vi "APU + 4 Digital Patterns.vi"() -> ()   [LabVIEW 2013]
uses:
  IP Source/Digital Pattern Generation/Load Input.ctl
  IP Source/Digital Pattern Generation/Input.ctl
  IP Source/Digital Pattern Generation/Settings.ctl
  IP Source/APU/Settings.ctl
  IP Source/APU/Input.ctl
  IP Source/APU/Output.ctl
  IP Source/Version Token.ctl
  IP Source/APU/Shared Settings.ctl
  <vilib>/Platform/TimedLoop/XDataNode/timing_clust.ctl
  <vilib>/Platform/TimedLoop/XDataNode/nitl_modes.ctl
  <vilib>/Platform/TimedLoop/XDataNode/wakeup.ctl
  <vilib>/rvi/DataTransferAndStorage/Container/Common/niFpgaContainerGetUniqueNameForEmu.vi
  <vilib>/rvi/DataTransferAndStorage/Container/Common/niFpgaContainerSetEmuInfo.vi
  <vilib>/rvi/eio/common/nirviEmuReportErrorAndStop.vi
  <vilib>/rvi/Emulation/niFpgaSctlEmulationGetInTimedLoop.vi
  <vilib>/rvi/Emulation/niFpgaEmulationReportErrorSimple.vi
  <vilib>/rvi/Emulation/niFpgaGetClockAttributes.vi
  <vilib>/rvi/Emulation/niFpgaCriticalErrorInLSC.vi
  <vilib>/rvi/eio/common/nirviEmuTemplateMethod_errors.vi
  <vilib>/Platform/TimedLoop/XDataNode/XDataNode.xnode
  <vilib>/rvi/LocalResourceManager/LocalResourceManager.xnode
  <vilib>/eio/EIONode/EIONode.xnode
  <vilib>/Platform/TimedLoop/XDataNode/XDNodeRunTimeDep.lvlib
  IP Source/Digital Pattern Generation/Digital Pattern Generation.lvlib
  IP Source/APU/APU.lvlib
  IP Source/Engine Simulation Toolkit.lvlib
panel:
  in  "shared settings.my apu":T1 {"start" format="%#.15g"}
  in  "go.my apu":bool
  in  "est.version":T2
  out "output.my apu":T3 caption="output"
  in  "input.my apu":T4={"desired speed"=0.0, "reset"=TRUE} caption="input"
  in  "settings.my apu":T5 caption="settings"
  in  "input.Pattern 3":T6
  in  "settings.Pattern 3":T7
  in  "input.Pattern 4":T6
  in  "settings.Pattern 4":T7
  in  "input.Pattern 2":T6
  in  "settings.Pattern 2":T7
  in  "settings.Pattern 1":T7
  in  "input.Pattern 1":T6
  in  "load input.Pattern 4":T8
  in  "load input.Pattern 3":T8
  in  "load input.Pattern 2":T8
  in  "load input.Pattern 1":T8
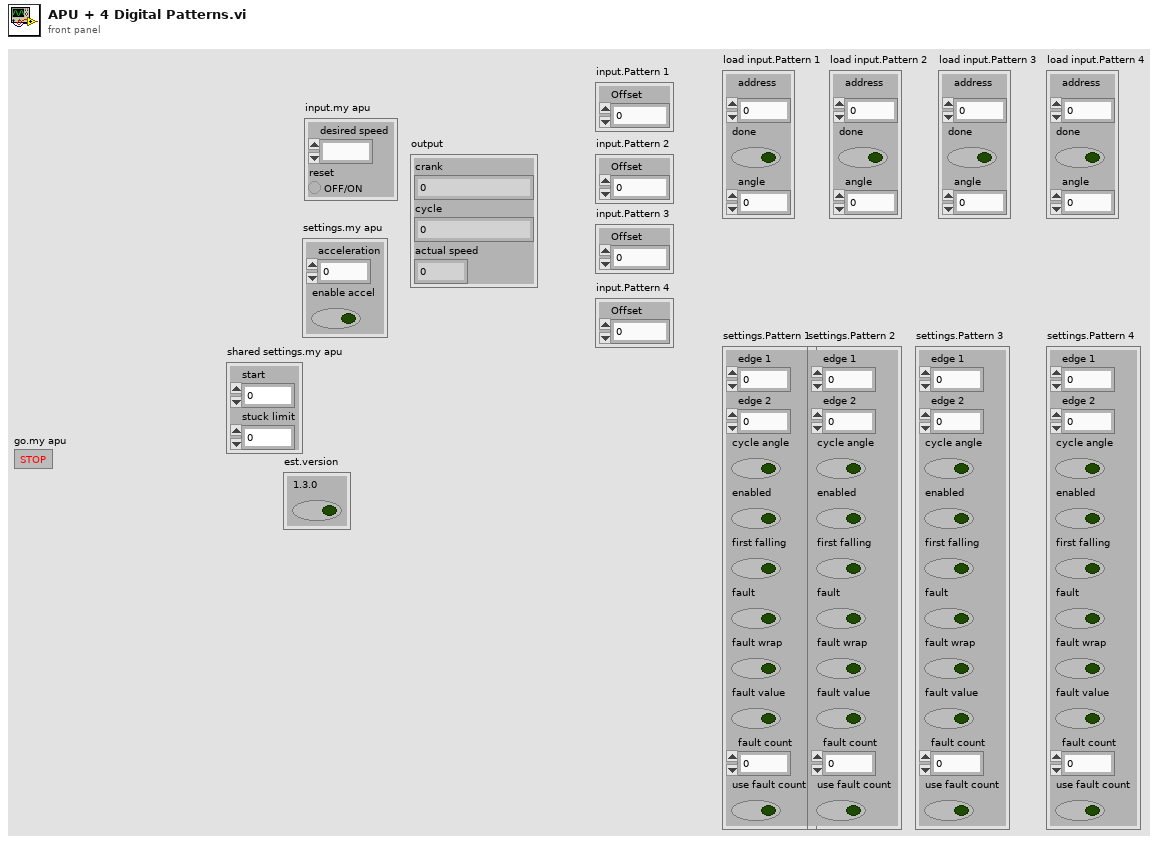
[diagram p1: front panel]
types:
  T1 = typedef "Engine Simulation Toolkit.lvlib/APU.lvlib/Shared Settings.ctl" = cluster{"start":fxp<+,17,17>, "stuck limit":fxp<+,18,18>}
  T2 = typedef "Engine Simulation Toolkit.lvlib/Version Token.ctl" = cluster{"1.3.0":bool}
  T3 = typedef "Engine Simulation Toolkit.lvlib/APU.lvlib/Output.ctl" = cluster{"crank":u16, "cycle":u16, "actual speed":fxp<+/-,23,2>}
  T4 = typedef "Engine Simulation Toolkit.lvlib/APU.lvlib/Input.ctl" = cluster{"desired speed":fxp<+/-,23,2>, "reset":bool}
  T5 = typedef "Engine Simulation Toolkit.lvlib/APU.lvlib/Settings.ctl" = cluster{"acceleration":fxp<+,18,-20>, "enable accel":bool}
  T6 = typedef "Engine Simulation Toolkit.lvlib/Digital Pattern Generation.lvlib/Input.ctl" = cluster{"Offset":i16}
  T7 = typedef "Engine Simulation Toolkit.lvlib/Digital Pattern Generation.lvlib/Settings.ctl" = cluster{"edge 1":u16, "edge 2":u16, "cycle angle":bool, "enabled":bool, "first falling":bool, "fault":bool, "fault wrap":bool, "fault value":bool, "fault count":fxp<+,4,4>, "use fault count":bool}
  T8 = typedef "Engine Simulation Toolkit.lvlib/Digital Pattern Generation.lvlib/Load Input.ctl" = cluster{"address":fxp<+,11,11>, "done":bool, "angle":u16}
  T9 = typedef "XDNodeRunTimeDep.lvlib/timing_clust.ctl" = cluster{"Expected End [f-1]":u64, "Actual End [f-1]":u64, "Finished Late? [f-1]":bool, "Expected End [i-1]":u64, "Actual End [i-1]":u64, "Finished Late? [i-1]":bool, "Expected Start [i]":u64, "Actual Start [i]":u64, "Expected Start [f]":u64, "Actual Start [f]":u64, "Source Name":string, "Structure Name":string, "Period":i64, "Deadline":i64, "Offset":i64, "Start":i64, "Priority":i32, "Timeout":i32, "Mode":T10, "Wakeup Reason":T11, "Error":errorcluster, "Source Type":string, "Secondary Source Type":string, "Global End Time":u64, "Global Start Time":u64, "Frame Duration":u64, "Iteration Duration":u64, "Assigned CPU":i32, "I/O Scan Engine Mode":u32}
  T10 = typedef "XDNodeRunTimeDep.lvlib/nitl_modes.ctl" = enum32{"No Change", "Process missed periods, maintain original phase", "Discard missed periods, maintain original phase", "Process missed periods, ignore original phase", "Discard missed periods, ignore original phase"}
  T11 = typedef "XDNodeRunTimeDep.lvlib/wakeup.ctl" = enum32{"Normal", "Aborted", "Asynchronous wakeup", "Timing source error", "Timed loop error", "Timeout"}
  T12 = typedef "Engine Simulation Toolkit.lvlib/Digital Pattern Generation.lvlib/Load Data.ctl" = cluster{"max address":fxp<+,11,11>, "memory":refnum<k21>}
  T13 = typedef "Engine Simulation Toolkit.lvlib/APU.lvlib/Register Bus.ctl" = cluster{"Speed":refnum<k21>, "Crank Angle":refnum<k21>, "Cycle Angle":refnum<k21>, "Crank Count":refnum<k21>, "Cycle Count":refnum<k21>, "1.25 MHz Counter":refnum<k21>, "Crank Rollover":refnum<k21>, "Cycle Rollover":refnum<k21>, "shared settings":T1}
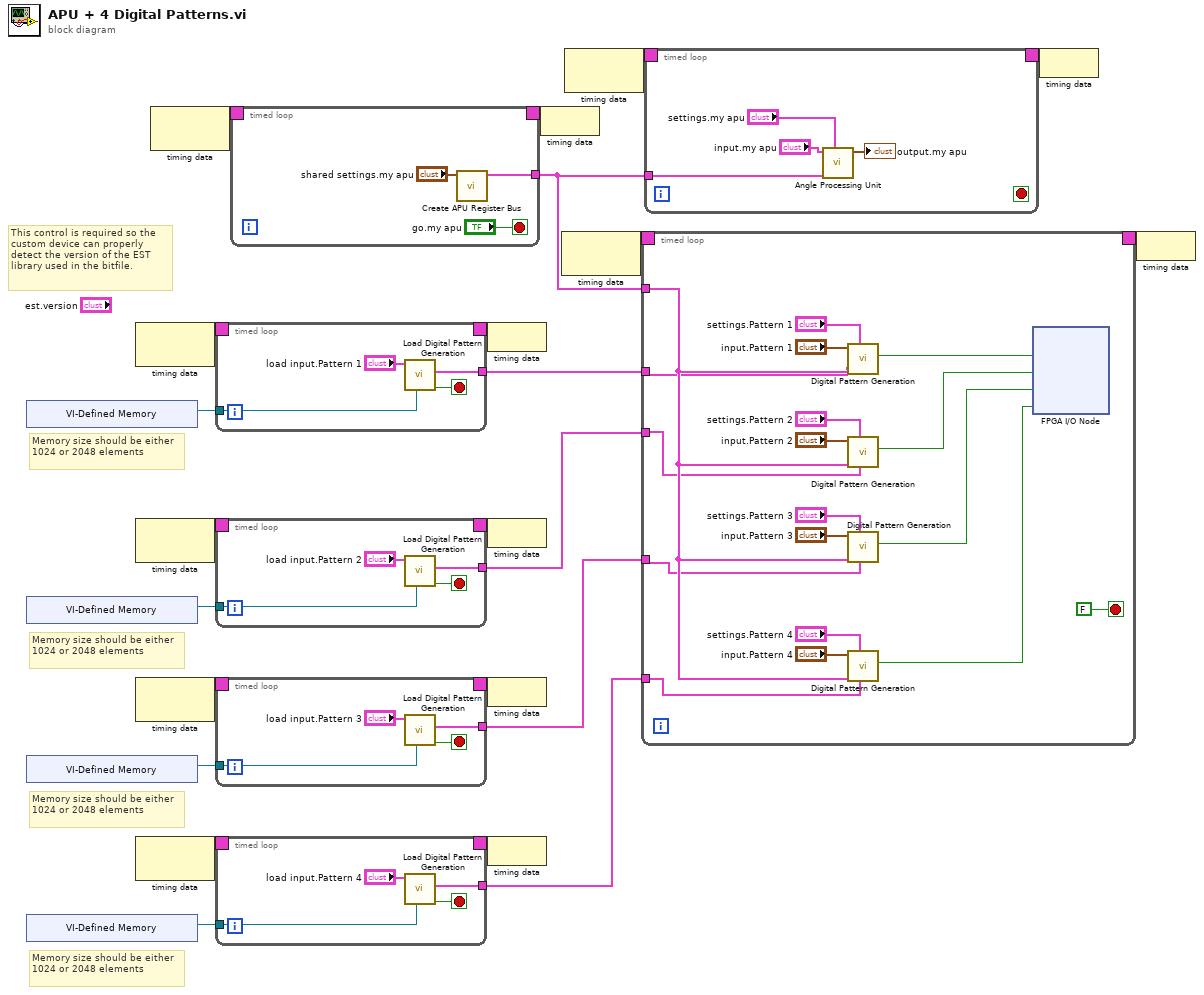
[diagram p0: block diagram]
diagram:
  # "This control is required so the custom device can properly detect the version of the EST library used in the bitfile."
  # "Memory size should be either 1024 or 2048 elements"
  # "Memory size should be either 1024 or 2048 elements"
  # "Memory size should be either 1024 or 2048 elements"
  # "Memory size should be either 1024 or 2048 elements"
  n1 = xnode "VI-Defined Memory"() -> ("Memory Out"=w21:refnum<k21>)
  n2 = xnode "VI-Defined Memory"() -> ("Memory Out"=w16:refnum<k21>)
  n3 = xnode "VI-Defined Memory"() -> ("Memory Out"=w13:refnum<k21>)
  n4 = xnode "VI-Defined Memory"() -> ("Memory Out"=w10:refnum<k21>)
  n5 = node-c288() -> (w23:T9)  [unwired: 1 in]
  n6 = node-c288() -> (w18:T9)  [unwired: 1 in]
  n7 = node-c288() -> (w15:T9)  [unwired: 1 in]
  n8 = node-c288() -> (w12:T9)  [unwired: 1 in]
  n9 = node-c288() -> (w3:T9)  [unwired: 1 in]
  n10 = timed-loop {
    timing: w23 -> [_]
    timing-out: [_] -> w22
    tunnel: w21 -> [w26]
    tunnel: [w25] -> w6
    stop <- w27 stop-if-true
    n11 = call "Load Digital Pattern Generation.vi"("memory"=w26, "load input.<user name>"="load input.Pattern 1") -> ("done"=w27:bool, "load data"=w25:T12)  [unwired: 8 in]
  }
  n12 = timed-loop {
    timing: w18 -> [_]
    timing-out: [_] -> w17
    tunnel: w16 -> [w32]
    tunnel: [w31] -> w9
    stop <- w33 stop-if-true
    n13 = call "Load Digital Pattern Generation.vi"("memory"=w32, "load input.<user name>"="load input.Pattern 2") -> ("done"=w33:bool, "load data"=w31:T12)  [unwired: 8 in]
  }
  n14 = timed-loop {
    timing: w15 -> [_]
    timing-out: [_] -> w14
    tunnel: w13 -> [w38]
    tunnel: [w37] -> w8
    stop <- w39 stop-if-true
    n15 = call "Load Digital Pattern Generation.vi"("memory"=w38, "load input.<user name>"="load input.Pattern 3") -> ("done"=w39:bool, "load data"=w37:T12)  [unwired: 8 in]
  }
  n16 = timed-loop {
    timing: w12 -> [_]
    timing-out: [_] -> w11
    tunnel: w10 -> [w44]
    tunnel: [w43] -> w7
    stop <- w45 stop-if-true
    n17 = call "Load Digital Pattern Generation.vi"("memory"=w44, "load input.<user name>"="load input.Pattern 4") -> ("done"=w45:bool, "load data"=w43:T12)  [unwired: 8 in]
  }
  n18 = timed-loop {
    timing: w3 -> [_]
    timing-out: [_] -> w2
    tunnel: [w50] -> w1
    stop <- "go.my apu" stop-if-true
    n19 = call "Create APU Register Bus.vi"("shared settings.<user name>"="shared settings.my apu") -> ("register bus"=w50:T13)  [unwired: 10 in]
  }
  n20 = node-c288(w22) -> ()
  n21 = node-c288(w17) -> ()
  n22 = node-c288(w14) -> ()
  n23 = node-c288(w11) -> ()
  n24 = node-c288(w2) -> ()
  n25 = node-c288() -> (w20:T9)  [unwired: 1 in]
  n26 = node-c288() -> (w5:T9)  [unwired: 1 in]
  n27 = timed-loop {
    tunnel: w1 -> [w57]
    timing: w20 -> [_]
    timing-out: [_] -> w19
    tunnel: w6 -> [w56]
    tunnel: w9 -> [w55]
    tunnel: w8 -> [w54]
    tunnel: w7 -> [w53]
    stop <- FALSE stop-if-true
    n28 = call "Digital Pattern Generation.vi"("load data"=w56, "settings.<user name>"="settings.Pattern 1", "register bus"=w57, "input.<user name>"="input.Pattern 1") -> ("digial output"=w62:bool)  [unwired: 7 in]
    n29 = call "Digital Pattern Generation.vi"("load data"=w55, "settings.<user name>"="settings.Pattern 2", "register bus"=w57, "input.<user name>"="input.Pattern 2") -> ("digial output"=w63:bool)  [unwired: 7 in]
    n30 = call "Digital Pattern Generation.vi"("load data"=w54, "settings.<user name>"="settings.Pattern 3", "register bus"=w57, "input.<user name>"="input.Pattern 3") -> ("digial output"=w64:bool)  [unwired: 7 in]
    n31 = call "Digital Pattern Generation.vi"("load data"=w53, "settings.<user name>"="settings.Pattern 4", "register bus"=w57, "input.<user name>"="input.Pattern 4") -> ("digial output"=w65:bool)  [unwired: 7 in]
    n32 = xnode "FPGA I/O Node"("DO0"=w62, "DO1"=w63, "DO2"=w64, "DO3"=w65) -> ()  [unwired: 4 in, 4 out]
  }
  n33 = timed-loop {
    timing: w5 -> [_]
    timing-out: [_] -> w4
    tunnel: w1 -> [w73]
    stop <- _ stop-if-true
    n34 = call "Angle Processing Unit.vi"("settings.<user name>"="settings.my apu", "register bus"=w73, "input.<user name>"="input.my apu") -> ("output.<user name>"=→"output.my apu":T3)  [unwired: 8 in]
  }
  n35 = node-c288(w4) -> ()
  n36 = node-c288(w19) -> ()
